vi "SetUpdateDelay.vi"(8 "error in (no error)":errorcluster, 10 "Update delay (ms)":u32, 11 "FolloWin in":refnum<class "FolloWin.lvclass">) -> (0 "error out":errorcluster, 3 "FolloWin out":refnum<class "FolloWin.lvclass">)   [LabVIEW 2023, in "FolloWin.lvclass"]
doc: "Sets the update rate of the FolloWin main cycle. \n\n-a low value will require more computer resources. \n-a high value will make window movement appear choppy."
uses:
  FolloWin.lvclass
  FolloWin.lvclass/FolloWin.ctl
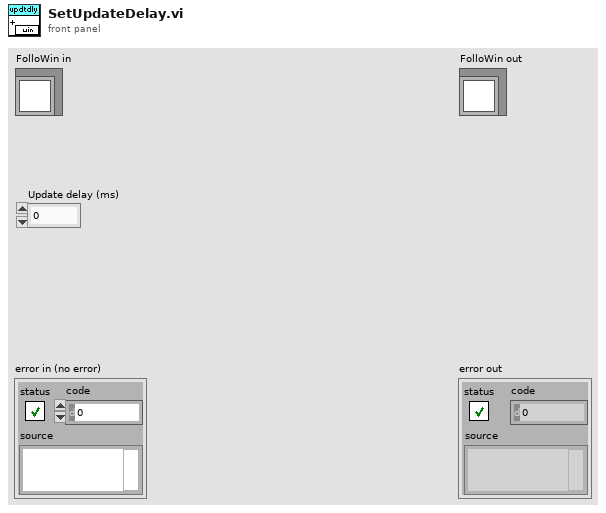
[diagram p1: front panel]
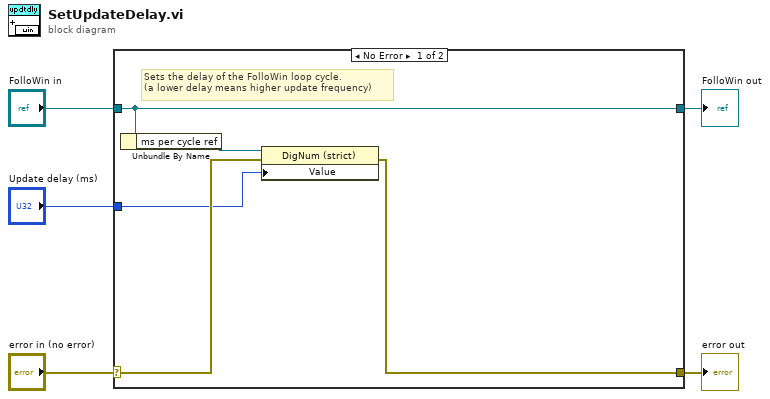
[diagram p0: block diagram]
diagram:
  n1 = case shown="No Error" "error in (no error)" {
    selector: "error in (no error)" -> [w8 w12]
    tunnel: [w7 w12] -> w4
    tunnel: [w10 w11] -> w2
    tunnel: "FolloWin in" -> [w10 w11]
    tunnel: "Update delay (ms)" -> [w6 _]
    frame No Error {
      # "Sets the delay of the FolloWin loop cycle. \n(a lower delay means higher update frequency)"
      n2 = Unbundle By Name(w10) -> ("ms per cycle ref"=w9:refnum<vi>)
      n3 = property on="Property Node" class="DigNum (strict)"(reference=w9, error in=w8, "Value"=w6) -> (error out=w7:errorcluster)  [unwired: 1 out]
    }
    frame Error {
    }
  }
  "error out" <- w4
  "FolloWin out" <- w2
